vi "openeod.vi"(0 "Byte Stream File in":refnum<file>, 1 "size (in bytes)":i64, 5 "error in (no error)":errorcluster) -> (6 "Wave":i16[][](array[numeric]), 7 "Wave Offset":i32[](array[numeric]), 8 "nchar":u8[](array[numeric]), 9 "polarity":i8[](array[numeric]), 10 "nWavepoints":u32[](array[numeric]), 11 "userdata":sgl[][](array[numeric]), 12 "Numeric":i32, 13 "nbytes":i8[](array[numeric]), 14 "Byte Stream File out":refnum<file>, 15 "ADrange":sgl[](array[numeric]), 16 "eodtext":string[](array[string]), 17 "srate":u32[](array[numeric]), 18 "nbits":i8[](array[numeric]), 19 "error out":errorcluster)   [LabVIEW 2013]
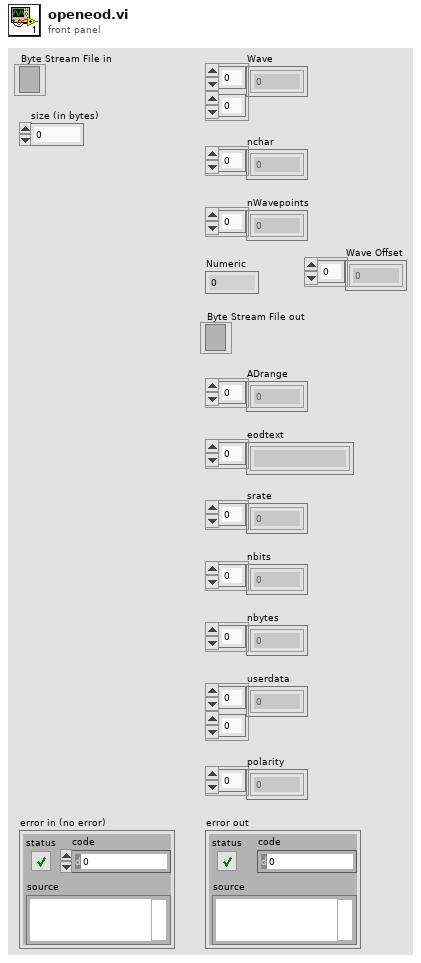
[diagram p1: front panel]
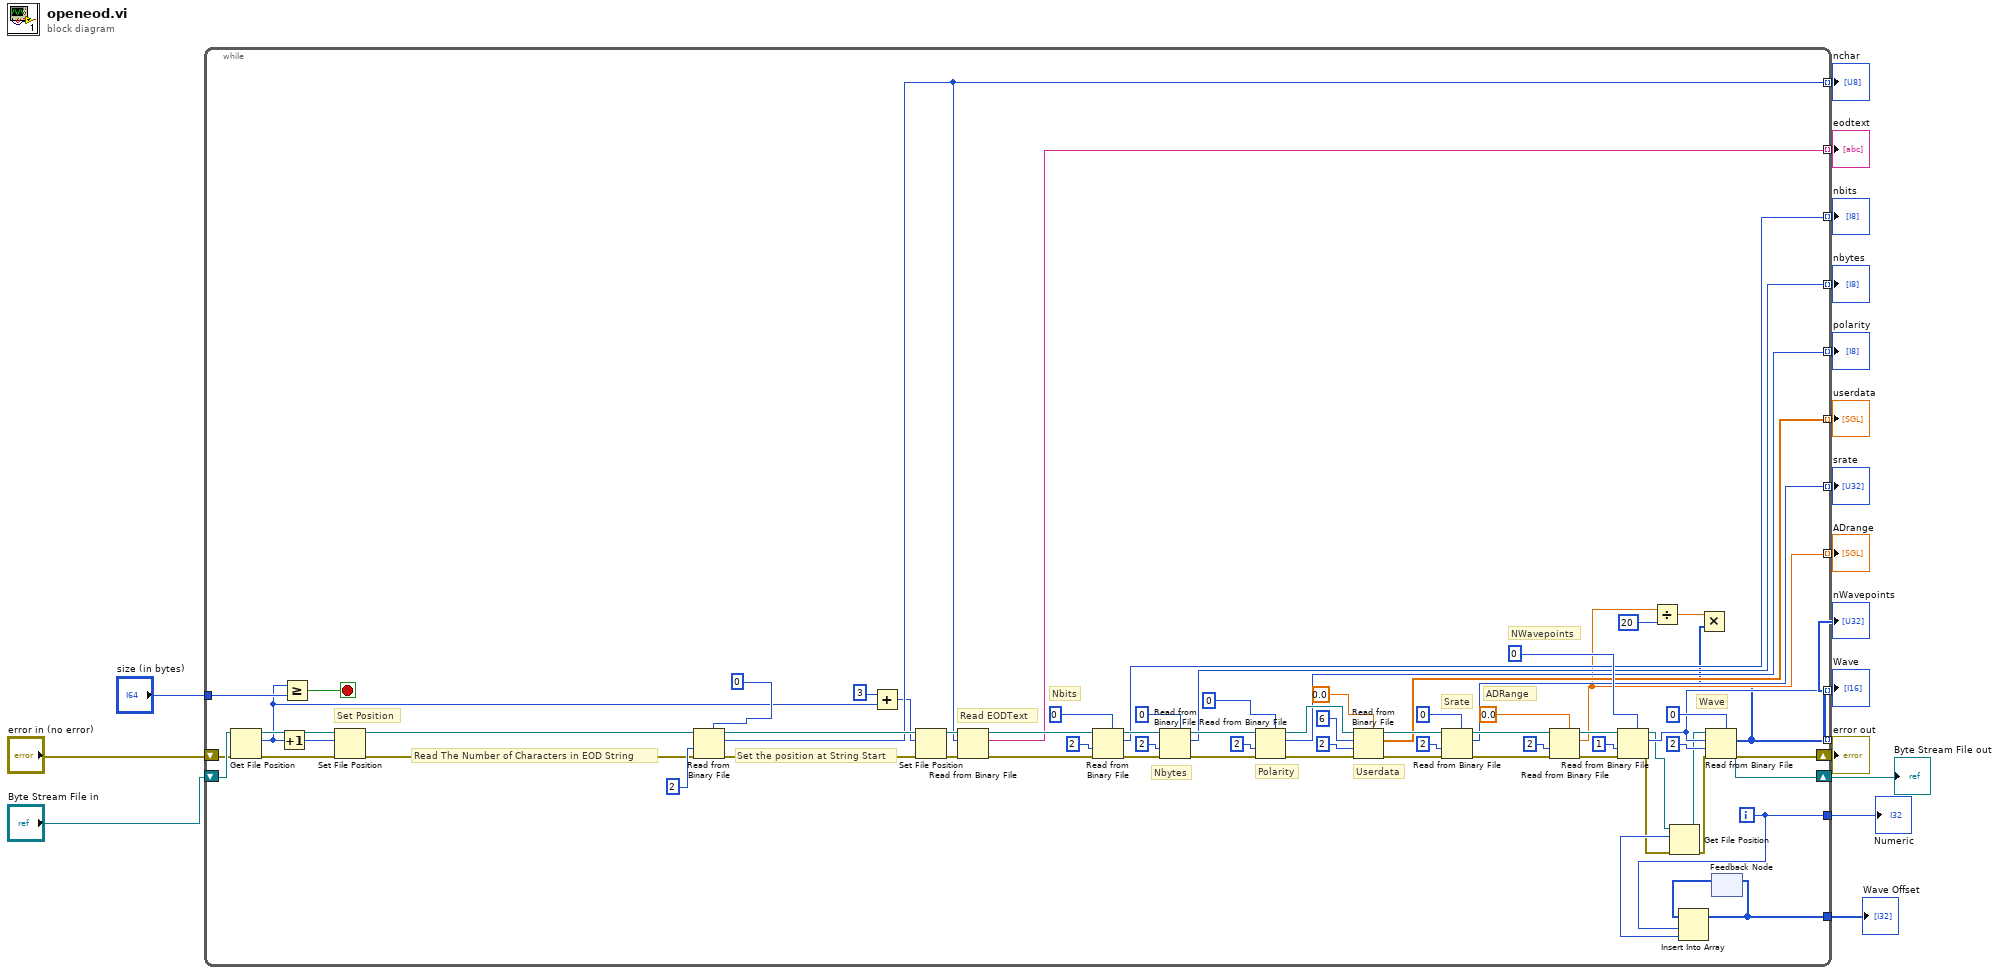
[diagram p0: block diagram]
diagram:
  n1 = while {
    tunnel: [w59] -> w2 mode=indexing
    tunnel: [w58] -> w3 mode=indexing
    tunnel: [w57] -> w4 mode=indexing
    tunnel: [w56] -> w5 mode=indexing
    tunnel: [w55] -> w6 mode=indexing
    tunnel: [w54] -> w7 mode=indexing
    tunnel: [w53] -> w8 mode=indexing
    tunnel: [w32] -> w9 mode=indexing
    tunnel: [w27] -> w11 mode=indexing
    tunnel: [w52] -> w10 mode=indexing
    shift-right: [w26] -> w15
    shift-left: "Byte Stream File in" -> [w40]
    shift-right: [w36] -> w16
    shift-left: "error in (no error)" -> [w37]
    tunnel: "size (in bytes)" -> [w33]
    tunnel: [w19] -> w14
    tunnel: [w18] -> w1
    i -> [w19]
    stop <- w41 stop-if-true
    # "Wave"
    # "NWavepoints"
    # "ADRange"
    # "Srate"
    # "Userdata"
    # "Polarity"
    # "Nbytes"
    # "Nbits"
    # "Read EODText"
    # "Set the position at String Start"
    # "Read The Number of Characters in EOD String"
    # "Set Position"
    n2 = Get File Position(4:w37, 7:w40) -> (0:w38:errorcluster, 2:w28:i64, 3:w39:refnum<file>)
    n3 = Increment(x=w28) -> (x+1=w29:i64)
    n4 = Greater Or Equal?(x=w28, y=w33) -> (x >= y?=w41:bool)
    n5 = Set File Position(offset (in bytes) (0)=w29, refnum=w39, error in=w38) -> (refnum out=w87:refnum<file>, error out=w51:errorcluster)  [unwired: 1 in]
    n6 = Read from Binary File(5:u8 0, 8:w51, 9:2, 11:w87) -> (0:w50:errorcluster, 2:w59:u8, 3:w86:refnum<file>)  [unwired: 2 in, 1 out]
    n7 = Add(x=3, y=w28) -> (x+y=w35:i64)
    n8 = Set File Position(offset (in bytes) (0)=w35, refnum=w86, error in=w50) -> (refnum out=w85:refnum<file>, error out=w49:errorcluster)  [unwired: 1 in]
    n9 = Read from Binary File(8:w49, 10:w59, 11:w85) -> (0:w48:errorcluster, 2:w58:string, 3:w84:refnum<file>)  [unwired: 3 in, 1 out]
    n10 = Read from Binary File(5:i8 0, 8:w48, 9:2, 11:w84) -> (0:w47:errorcluster, 2:w57:i8, 3:w61:refnum<file>)  [unwired: 2 in, 1 out]
    n11 = Read from Binary File(5:i8 0, 8:w47, 9:2, 11:w61) -> (0:w46:errorcluster, 2:w56:i8, 3:w62:refnum<file>)  [unwired: 2 in, 1 out]
    n12 = Read from Binary File(5:i8 0, 8:w46, 9:2, 11:w62) -> (0:w45:errorcluster, 2:w55:i8, 3:w60:refnum<file>)  [unwired: 2 in, 1 out]
    n13 = Read from Binary File(5:sgl 0.0, 8:w45, 9:2, 10:6, 11:w60) -> (0:w44:errorcluster, 2:w54:sgl[], 3:w81:refnum<file>)  [unwired: 1 in, 1 out]
    n14 = Read from Binary File(5:u32 0, 8:w44, 9:2, 11:w81) -> (0:w43:errorcluster, 2:w53:u32, 3:w73:refnum<file>)  [unwired: 2 in, 1 out]
    n15 = Read from Binary File(5:sgl 0.0, 8:w43, 9:2, 11:w73) -> (0:w42:errorcluster, 2:w32:sgl, 3:w68:refnum<file>)  [unwired: 2 in, 1 out]
    n16 = Read from Binary File(5:u32 0, 8:w42, 9:1, 11:w68) -> (0:w21:errorcluster, 2:w52:u32, 3:w23:refnum<file>)  [unwired: 2 in, 1 out]
    n17 = Divide(x=w32, y=20) -> (x/y=w30:sgl)
    n18 = Get File Position(4:w21, 7:w23) -> (0:w20:errorcluster, 2:w25:i64, 3:w22:refnum<file>)
    n19 = Read from Binary File(5:i16 0, 8:w20, 9:2, 10:w52, 11:w22) -> (0:w36:errorcluster, 2:w27:i16[], 3:w26:refnum<file>)  [unwired: 1 in, 1 out]
    n20 = Multiply(x=w30, y=w27) -> ()  [unwired: 1 out]
    n21 = feedback #1() -> (w24:i64[])  [unwired: 1 in]
    n22 = Insert Into Array(array=w24, index=w19, new element=w25) -> (w18:i64[])
    n23 = feedback-in #1(w18) -> ()
  }
  "error out" <- w16
  "Byte Stream File out" <- w15
  "Numeric" <- w14
  "Wave" <- w11
  "nWavepoints" <- w10
  "ADrange" <- w9
  "srate" <- w8
  "userdata" <- w7
  "polarity" <- w6
  "nbytes" <- w5
  "nbits" <- w4
  "eodtext" <- w3
  "nchar" <- w2
  "Wave Offset" <- w1
